vi "getBounds.vi"(0 "reference":refnum<class "PointNode.lvclass">, 5 "error in (no error)":errorcluster) -> (14 "reference out":refnum<class "PointNode.lvclass">, 15 "bounds":T1 {"height" format="%.2f"; "width" format="%.2f"; "y" format="%.2f"; "x" format="%.2f"}, 19 "error out":errorcluster)   [LabVIEW 2020, in "PointNode.lvclass"]
doc: "public Rectangle2D getBounds()"
uses:
  <resource>/Framework/Providers/Open_GDS/UML/PointNode_class/PointNode.lvclass
  <resource>/Framework/Providers/Open_GDS/UML/General/Rectangle/Rectangle Rectangle2D.ctl
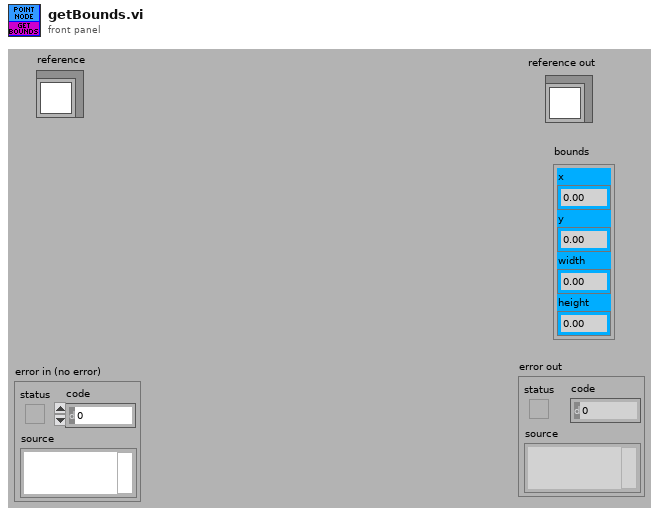
[diagram p1: front panel]
types:
  T1 = typedef "Rectangle Rectangle2D.ctl" = cluster{"x":dbl, "y":dbl, "width":dbl, "height":dbl}
  T2 = typedef "PointNode.lvclass/ObjectAttributes.ctl" = cluster{"point":T3}
  T3 = typedef "Point Point2D.ctl" = cluster{"x":dbl, "y":dbl}
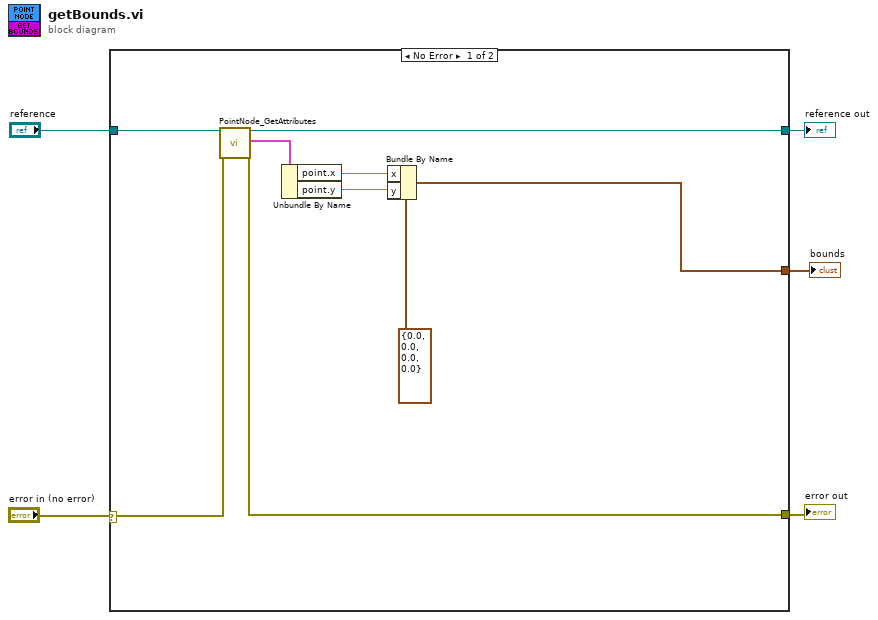
[diagram p0: block diagram]
diagram:
  n1 = case shown="No Error" "error in (no error)" {
    selector: "error in (no error)" -> [w7 w15]
    tunnel: "reference" -> [w14 w16]
    tunnel: [w13 w15] -> w4
    tunnel: [w12 w16] -> w3
    tunnel: [w11 _] -> w1
    frame No Error {
      n2 = call <resource>:"PointNode_GetAttributes.vi"("reference in"=w14, "error in (no error)"=w7) -> ("reference out"=w12:refnum<class "PointNode.lvclass">, "Data"=w6:T2, "error out"=w13:errorcluster)  [unwired: 1 in, 14 out]
      n3 = Unbundle By Name(w6) -> ("point.x"=w9:dbl, "point.y"=w8:dbl)
      n4 = Bundle By Name(cluster=T1 {"x"=0.0, "y"=0.0, "width"=0.0, "height"=0.0} ("bounds"), "x"=w9, "y"=w8) -> (w11:T1)
    }
    frame Error {
    }
  }
  "reference out" <- w3
  "error out" <- w4
  "bounds" <- w1
